vi "LV_XP_Controller.vi"() -> ()   [LabVIEW 2014]
panel:
  in  "Tab Control":enum32{"Roll", "Pitch", "Airspeed"}(tab)
  out "Output\nComponents":cluster{sgl, sgl, sgl, sgl, sgl, sgl}(graph)
  out "Roll \nChart":cluster{sgl, "Setpoint out":sgl}(graph)
  in  "Enable":T1
  in  "Gains":cluster{"P":sgl, "I":sgl, "D":sgl}={"P"=0.1, "I"=0.1, "D"=0.1}
  in  "Roll\nSetpoint":sgl(slide) scale=-45.0..45.0
  in  "Setpoint\nSource":T2(radio)
  in  "Signal\nParameters":T3
  in  "Pitch\nSetpoint":sgl(slide) scale=-15.0..15.0
  in  "Setpoint\nSource":T2(radio)
  out "Pitch Chart":cluster{sgl, "Pitch Setpoint":sgl}(graph)
  in  "Signal\nParameters":T3
  in  "Gains":cluster{"P":sgl, "I":sgl, "D":sgl}={"P"=0.1, "I"=0.1, "D"=0.1}
  in  "Enable":T1
  out "Output\nComponents\nChart":cluster{sgl, sgl, sgl, sgl, sgl, sgl}(graph)
  out "Airspeed\nChart":cluster{sgl, "Pitch Setpoint":sgl}(graph)
  in  "Airspeed \nSetpoint":sgl(slide) scale=0.0..300.0
  in  "Setpoint\nSource":T2(radio)
  in  "Signal\nParameters":T3
  out "Output\nComponents":cluster{sgl, sgl, sgl, sgl, sgl, sgl}(graph)
  in  "Enable":T1
  in  "Gains":cluster{"P":sgl, "I":sgl, "D":sgl}={"P"=0.1, "I"=0.1, "D"=0.1}
  in  "Heading \nHold":bool
  in  "stop":bool
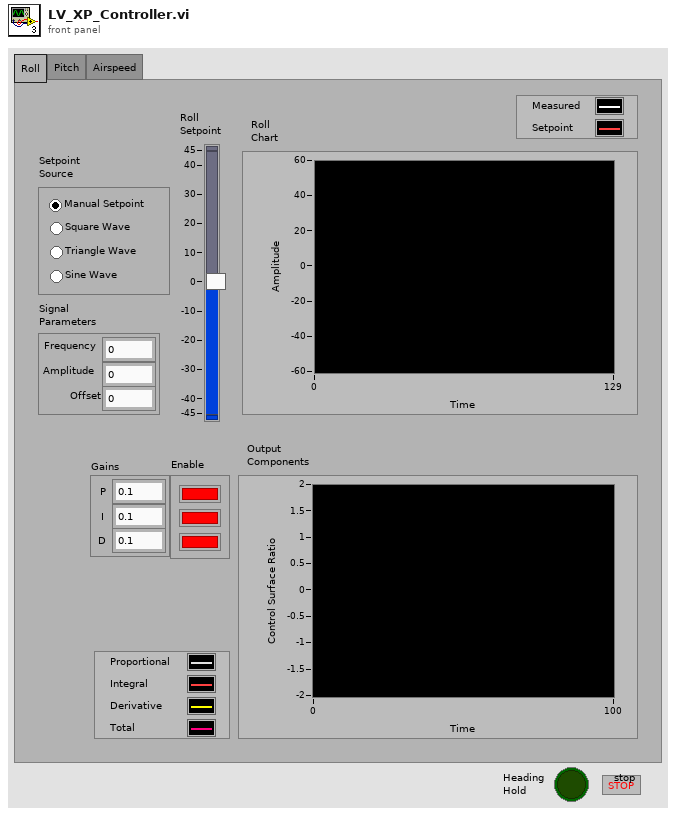
[diagram p1: front panel]
types:
  T1 = cluster{"P Enable":bool, "I Enable":bool, "D Enable":bool}
  T2 = enum32{"Manual Setpoint", "Square Wave", "Triangle Wave", "Sine Wave"}
  T3 = cluster{"Frequency":sgl, "Amplitude":sgl, "Offset":sgl}
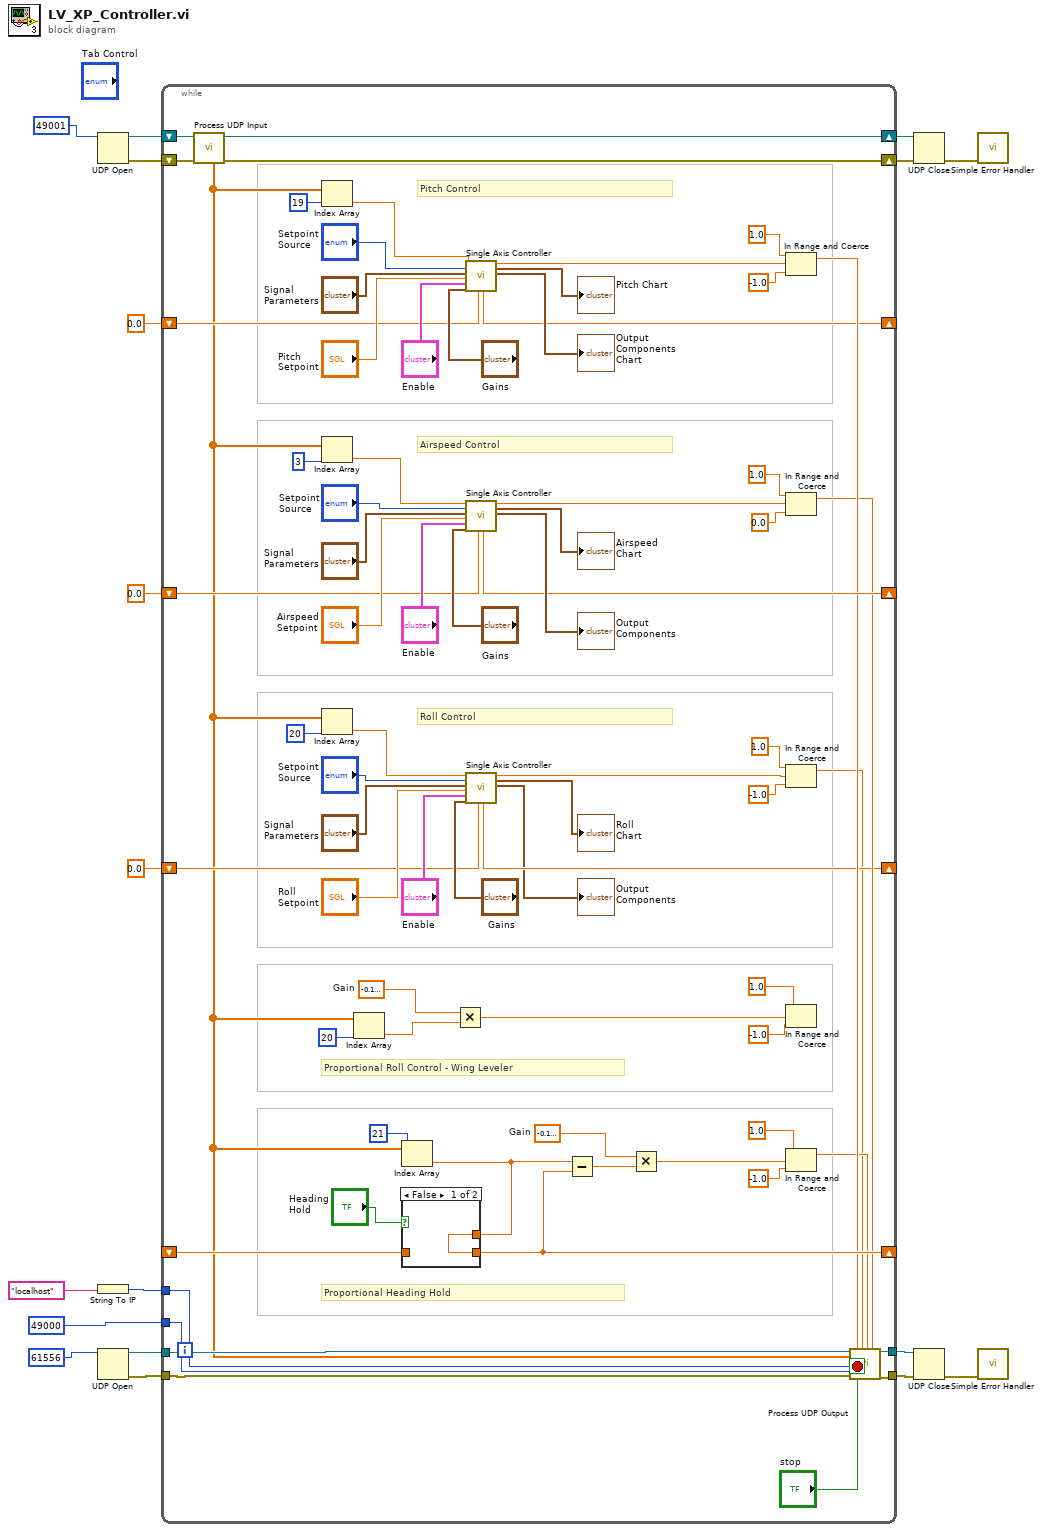
[diagram p0: block diagram]
diagram:
  n1 = UDP Open(11:u16 49001 ("port")) -> (port=w16:refnum<k16>, 0:w17:errorcluster)  [unwired: 4 in, 1 out]
  n2 = String To IP(1:"localhost") -> (0:w5:u32)
  n3 = UDP Open(11:u16 61556 ("port")) -> (port=w9:refnum<k16>, 0:w10:errorcluster)  [unwired: 4 in, 1 out]
  n4 = while {
    shift-right: [w88] -> w15
    shift-left: w17 -> [w92]
    shift-right: [w90] -> w14
    shift-left: w16 -> [w91]
    tunnel: [w86] -> w11
    tunnel: w10 -> [w85]
    tunnel: w9 -> [w84]
    tunnel: [w83] -> w8
    tunnel: w5 -> [w66]
    tunnel: 49000 -> [w65]
    shift-right: [w74] -> _
    shift-left: _ -> [w73]
    shift-right: [w21] -> _
    shift-left: sgl 0.0 ("Integral Out") -> [w55]
    shift-right: [w54] -> _
    shift-left: 0.0 ("Integral Out") -> [w53]
    shift-right: [w32] -> _
    shift-left: 0.0 ("Integral Out") -> [w31]
    stop <- "stop" stop-if-true
    w78 = sgl -0.1  # Gain
    w80 = sgl -0.1  # Gain
    # "Roll Control"
    # "Airspeed Control"
    # "Pitch Control"
    # "Proportional Heading Hold"
    # "Proportional Roll Control - Wing Leveler"
    n5 = call "Process UDP Input.vi"("error in (no error)"=w92, "UDP Network Connection in"=w91) -> ("error out"=w88:errorcluster, "Data From XPlane"=w24:sgl[], "UDP Network Connection out"=w90:refnum<k16>)  [unwired: 7 in]
    n6 = Index Array(array=w24, index=19) -> (element=w20:sgl)
    n7 = Index Array(array=w24, index=3) -> (element=w19:sgl)
    n8 = Index Array(array=w24, index=20) -> (element=w23:sgl)
    n9 = Index Array(array=w24, index=20) -> (element=w81:sgl)
    n10 = Index Array(array=w24, index=21) -> (element=w75:sgl)
    n11 = case shown="False" "Heading \nHold" {
      tunnel: w75 -> [w93 _]
      tunnel: [w93 w94] -> w74
      tunnel: w73 -> [_ w94]
      frame False {
      }
      frame True {
      }
    }
    n12 = Multiply(x=w80, y=w81) -> (x*y=w40:sgl)
    n13 = call "Single Axis Controller.vi"("Measured Value"=w20, "Setpoint\nSource"="Setpoint\nSource", "Signal\nParameters"="Signal\nParameters", "Manual\nSetpoint"="Pitch\nSetpoint", "Enable"="Enable", "Gains"="Gains", "Integral In"=w55) -> ("Integral Out"=w21:sgl, "Controller \nOutput"=w52:sgl, "Sepoint \nChart"=→"Pitch Chart":cluster{sgl, "Setpoint out":sgl}, "Output\nComponents\nChart"=→"Output\nComponents\nChart":cluster{sgl, sgl, sgl, sgl, sgl, sgl})  [unwired: 8 in, 1 out]
    n14 = call "Single Axis Controller.vi"("Measured Value"=w19, "Setpoint\nSource"="Setpoint\nSource", "Signal\nParameters"="Signal\nParameters", "Manual\nSetpoint"="Airspeed \nSetpoint", "Enable"="Enable", "Gains"="Gains", "Integral In"=w53) -> ("Integral Out"=w54:sgl, "Controller \nOutput"=w42:sgl, "Sepoint \nChart"=→"Airspeed\nChart":cluster{sgl, "Setpoint out":sgl}, "Output\nComponents\nChart"=→"Output\nComponents":cluster{sgl, sgl, sgl, sgl, sgl, sgl})  [unwired: 8 in, 1 out]
    n15 = call "Single Axis Controller.vi"("Measured Value"=w23, "Setpoint\nSource"="Setpoint\nSource", "Signal\nParameters"="Signal\nParameters", "Manual\nSetpoint"="Roll\nSetpoint", "Enable"="Enable", "Gains"="Gains", "Integral In"=w31) -> ("Integral Out"=w32:sgl, "Controller \nOutput"=w25:sgl, "Sepoint \nChart"=→"Roll \nChart":cluster{sgl, "Setpoint out":sgl}, "Output\nComponents\nChart"=→"Output\nComponents":cluster{sgl, sgl, sgl, sgl, sgl, sgl})  [unwired: 8 in, 1 out]
    n16 = Subtract(x=w75, y=w74) -> (x-y=w77:sgl)
    n17 = Multiply(x=w78, y=w77) -> (x*y=w39:sgl)
    n18 = In Range and Coerce(upper limit=sgl 1.0, x=w52, lower limit=sgl -1.0) -> (coerced(x)=w51:sgl)  [unwired: 1 out]
    n19 = In Range and Coerce(upper limit=sgl 1.0, x=w42, lower limit=sgl 0.0) -> (coerced(x)=w41:sgl)  [unwired: 1 out]
    n20 = In Range and Coerce(upper limit=sgl 1.0, x=w25, lower limit=sgl -1.0) -> (coerced(x)=w22:sgl)  [unwired: 1 out]
    n21 = In Range and Coerce(upper limit=sgl 1.0, x=w40, lower limit=sgl -1.0) -> ()  [unwired: 2 out]
    n22 = In Range and Coerce(upper limit=sgl 1.0, x=w39, lower limit=sgl -1.0) -> (coerced(x)=w38:sgl)  [unwired: 1 out]
    n23 = call "Process UDP Output.vi"("UDP Network Connection in"=w84, "Data From Xplane"=w24, "IP Address"=w66, "Port"=w65, "error in (no error)"=w85, "Elevator"=w51, "Aileron"=w22, "Rudder"=w38, "Throttle"=w41) -> ("UDP Network \nConnection out"=w83:refnum<k16>, "error out"=w86:errorcluster)  [unwired: 9 in]
  }
  n24 = UDP Close(connection ID=w14, 8:w15) -> (error out=w13:errorcluster)  [unwired: 1 out]
  n25 = UDP Close(connection ID=w8, 8:w11) -> (error out=w12:errorcluster)  [unwired: 1 out]
  n26 = call <vilib>:"Simple Error Handler.vi"("error in (no error)"=w13) -> ()  [unwired: 4 in, 5 out]
  n27 = call <vilib>:"Simple Error Handler.vi"("error in (no error)"=w12) -> ()  [unwired: 4 in, 5 out]
